vi "Adquirir Imagen.vi"(8 "error in (no error)":errorcluster, 11 "Simulada in":refnum<class "Simulada.lvclass">) -> (0 "error out":errorcluster, 2 "Imagen":T1, 3 "Simulada out":refnum<class "Simulada.lvclass">)   [LabVIEW 2020, in "Simulada.lvclass"]
uses:
  Simulada.lvclass
  C:/Users/enoea/Desktop/DemoOOP/Clases/Abstracta/Camara/Camara.lvclass
  <vilib>/vision/Image Controls.llb/IMAQ Image.ctl
  Simulada.lvclass/Simulada.ctl
  Abstracta/Camara/Camara.lvclass/Camara.ctl
  Read RutaImagenes.vi
  Abstracta/Camara/Read New Image.vi
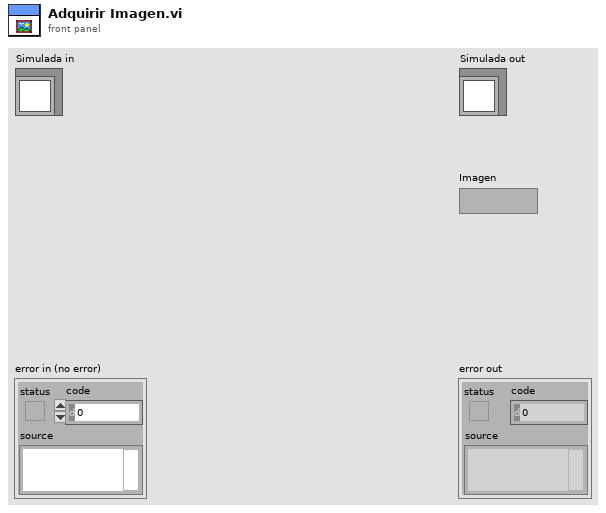
[diagram p1: front panel]
types:
  T1 = typedef "IMAQ Image.ctl" = refnum<image>
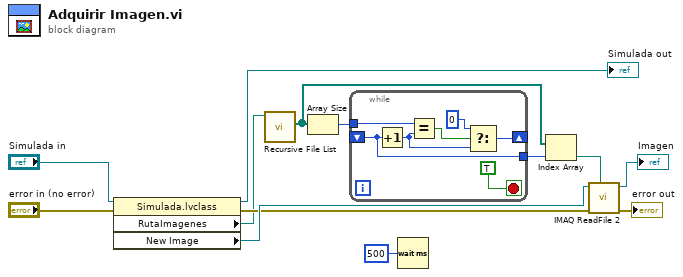
[diagram p0: block diagram]
diagram:
  n1 = property class="Simulada.lvclass"(reference="Simulada in", error in="error in (no error)") -> (reference out=→"Simulada out":refnum<class "Simulada.lvclass">, error out=w7:errorcluster, "RutaImagenes"=w2:path, "New Image"=w8:T1)
  n2 = call <vilib>:"Recursive File List.vi"("Folder Path"=w2) -> ("All Files in Dir"=w5:path[])  [unwired: 6 in, 4 out]
  n3 = Array Size(array=w5) -> (size(s)=w4:i32)
  n4 = while {
    tunnel: w4 -> [w20]
    shift-right: [w16] -> _
    shift-left: _ -> [w14]
    tunnel: [w14] -> w3
    stop <- TRUE stop-if-true
    n5 = Increment(x=w14) -> (x+1=w18:i32)
    n6 = Equal?(x=w20, y=w18) -> (x = y?=w19:bool)
    n7 = Select(t=0, s=w19, f=w18) -> (s? t:f=w16:i32)
  }
  n8 = Wait (ms)(milliseconds to wait=u32 500) -> ()  [unwired: 1 out]
  n9 = Index Array(array=w5, index=w3) -> (element=w9:path)
  n10 = call "IMAQ ReadFile 2"("File Path"=w9, "error in (no error)"=w7, "Image"=w8) -> ("error out"=→"error out":errorcluster, "Image Out"=→"Imagen":T1)  [unwired: 4 in, 3 out]
